vi "Pre-Uninstall Custom Action.vi"(10 "Variant":variant) -> (0 "error out":errorcluster)   [LabVIEW 2020]
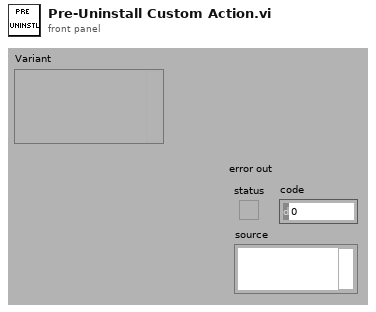
[diagram p1: front panel]
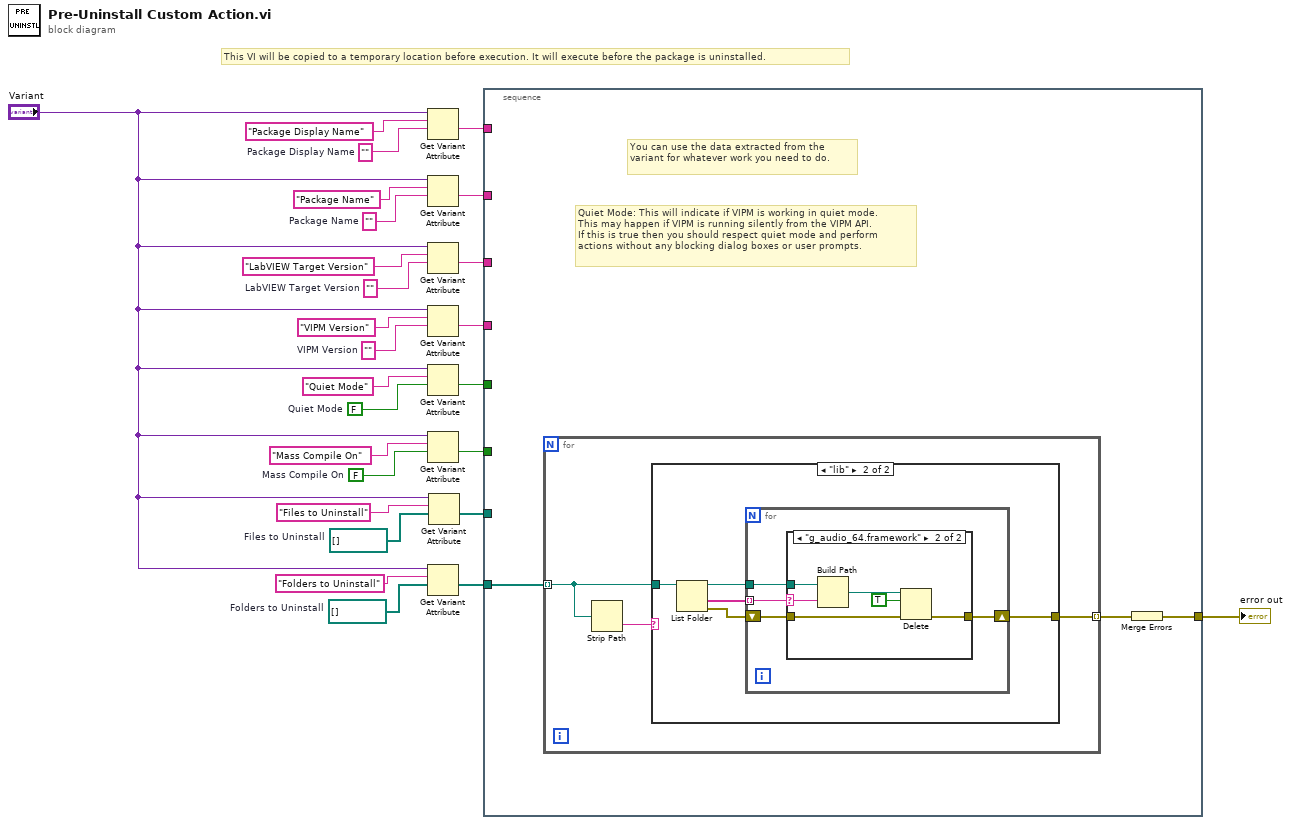
[diagram p0: block diagram]
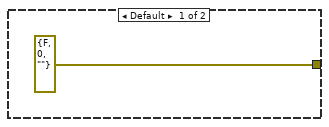
[diagram p2: hidden frame]
diagram:
  w4 = path[] []  # Folders to Uninstall
  w8 = path[] []  # Files to Uninstall
  w9 = FALSE  # Mass Compile On
  w10 = ""  # Package Display Name
  w17 = FALSE  # Quiet Mode
  w20 = ""  # VIPM Version
  w22 = ""  # LabVIEW Target Version
  w24 = ""  # Package Name
  # "This VI will be copied to a temporary location before execution. It will execute before the package is uninstalled."
  n1 = Get Variant Attribute(Variant="Variant", name="Package Display Name", default value (empty Variant)=w10) -> (value=w16:string)  [unwired: 1 in, 3 out]
  n2 = Get Variant Attribute(Variant="Variant", name="Package Name", default value (empty Variant)=w24) -> (value=w15:string)  [unwired: 1 in, 3 out]
  n3 = Get Variant Attribute(Variant="Variant", name="LabVIEW Target Version", default value (empty Variant)=w22) -> (value=w14:string)  [unwired: 1 in, 3 out]
  n4 = Get Variant Attribute(Variant="Variant", name="VIPM Version", default value (empty Variant)=w20) -> (value=w13:string)  [unwired: 1 in, 3 out]
  n5 = Get Variant Attribute(Variant="Variant", name="Quiet Mode", default value (empty Variant)=w17) -> (value=w12:bool)  [unwired: 1 in, 3 out]
  n6 = Get Variant Attribute(Variant="Variant", name="Mass Compile On", default value (empty Variant)=w9) -> (value=w11:bool)  [unwired: 1 in, 3 out]
  n7 = Get Variant Attribute(Variant="Variant", name="Folders to Uninstall", default value (empty Variant)=w4) -> (value=w3:path[])  [unwired: 1 in, 3 out]
  n8 = Get Variant Attribute(Variant="Variant", name="Files to Uninstall", default value (empty Variant)=w8) -> (value=w6:path[])  [unwired: 1 in, 3 out]
  n9 = stacked-sequence {
    tunnel: w16 -> [_]
    tunnel: w15 -> [_]
    tunnel: w14 -> [_]
    tunnel: w13 -> [_]
    tunnel: w12 -> [_]
    tunnel: w11 -> [_]
    tunnel: w6 -> [_]
    tunnel: w3 -> [w29]
    tunnel: [w27] -> w1
    frame #0 {
      # "Quiet Mode: This will indicate if VIPM is working in quiet mode.\nThis may happen if VIPM is running silently from the VIPM API.\nIf this is true then you should respect quiet mode and perform\nactions without any blocking dialog boxes or user prompts."
      # "You can use the data extracted from the variant for whatever work you need to do."
      n10 = for {
        tunnel: w29 -> [w32] mode=indexing
        tunnel: [w31] -> w28 mode=indexing
        n11 = Strip Path(path=w32) -> (name=w30:string)  [unwired: 1 out]
        n12 = case shown="\"lib\"" w30 {
          tunnel: w32 -> [_ w36]
          tunnel: [errorcluster {"status"=FALSE, "code"=0, "source"=""} ("error out") w35] -> w31
          frame Default {
          }
          frame "lib" {
            n13 = List Folder(path=w36) -> (path out=w38:path, folder names=w34:string[], error out=w37:errorcluster)  [unwired: 3 in, 1 out]
            n14 = for {
              tunnel: w38 -> [w39]
              shift-right: [w42] -> w35
              shift-left: w37 -> [w41]
              tunnel: w34 -> [w40] mode=indexing
              n15 = case shown="\"g_audio_64.framework\"" w40 {
                selector: w40 -> [_ w49]
                tunnel: w41 -> [w43 w46]
                tunnel: [w43 w48] -> w42
                tunnel: w39 -> [_ w47]
                frame Default {
                }
                frame "g_audio_64.framework" {
                  n16 = Build Path(base path=w47, name or relative path=w49) -> (appended path=w45:path)
                  n17 = Delete(path (use dialog)=w45, entire hierarchy (F)=TRUE, error in=w46) -> (error out=w48:errorcluster)  [unwired: 2 in, 2 out]
                }
              }
            }
          }
        }
      }
      n18 = Merge Errors(w28) -> (w27:errorcluster)
    }
  }
  "error out" <- w1
